vi "Booleanos.vi"() -> ()   [LabVIEW 2020]
panel:
  out "OR 2":bool
  out "NOT":bool
  out "XOR":bool
  out "OR":bool
  out "AND":bool
  in  "Boton2":bool
  in  "Boton1":bool
  # "Compuertas Logicas"
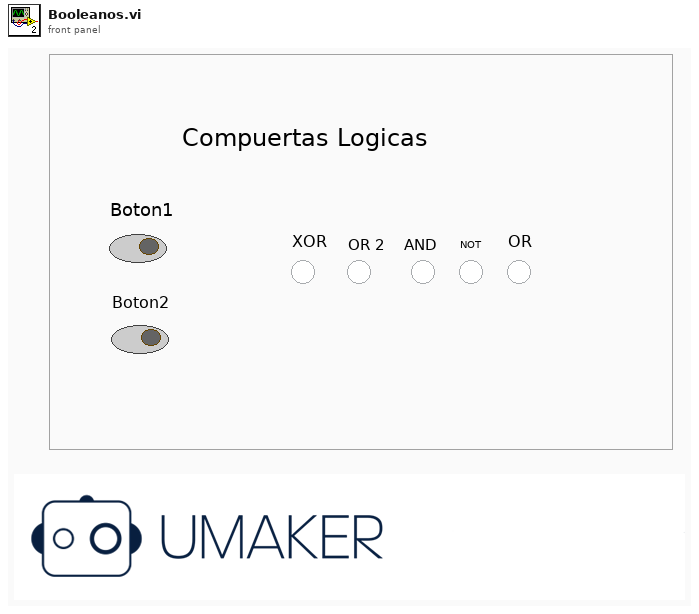
[diagram p1: front panel]
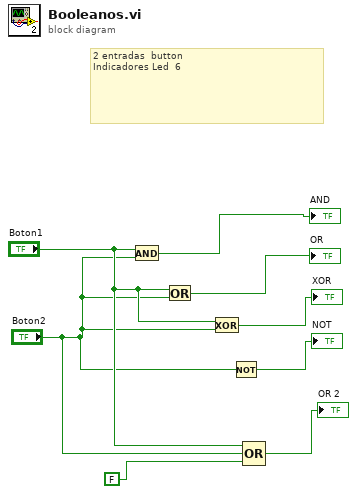
[diagram p0: block diagram]
diagram:
  # "2 entradas  button \nIndicadores Led  6"
  n1 = And(x="Boton1", y="Boton2") -> (x .and. y?=→"AND":bool)
  n2 = Or(x="Boton1", y="Boton2") -> (x .or. y?=→"OR":bool)
  n3 = Exclusive Or(1:"Boton2", 2:"Boton1") -> (0:→"XOR":bool)
  n4 = Not(x="Boton2") -> (.not. x?=→"NOT":bool)
  n5 = Compound Arithmetic op=OR("Boton1", "Boton2", FALSE) -> (→"OR 2":bool)
